vi "Read Waveform (Multiple).vi"(8 "error in (no error)":errorcluster, 9 "Maximum Time (10000 ms)":u32=10000, 10 "Channels":u16[](array[ring])=[1, 2] items=["Channel 1"=1, "Channel 2"=2], 11 "VISA resource name":refnum<visa-resource-name>) -> (0 "error out":errorcluster, 2 "Waveform Data":waveform(dbl)[](graph), 3 "VISA resource name out":refnum<visa-resource-name>)   [LabVIEW 2013, in "Template - Scope.lvlib"]
doc: "Initiates an acquisition on all channels that you enabled with the Configure Channel VI. The VI waits for the acquisition to complete and returns the waveform for the <B>Source Channel</B> you specified. If the oscilloscope did not complete the acquisition within the time period you specify with the <B>Timeout</B> control, the VI returns a timeout error. A common cause for a timeout error is the acquisition was not triggered. For example, the trigger level is out of range of the waveform. \n\n<B>Note:</B> If your instrument does not support auto compensation for probe attenuation, you may need to adjust the scaling of the waveform data accordingly. This is handled automatically in the Configure Channel VI or can be done manually by multiplying the waveform data by the probe attenuation."
uses:
  <instrlib>/_Template - Scope/Template - Scope.lvlib
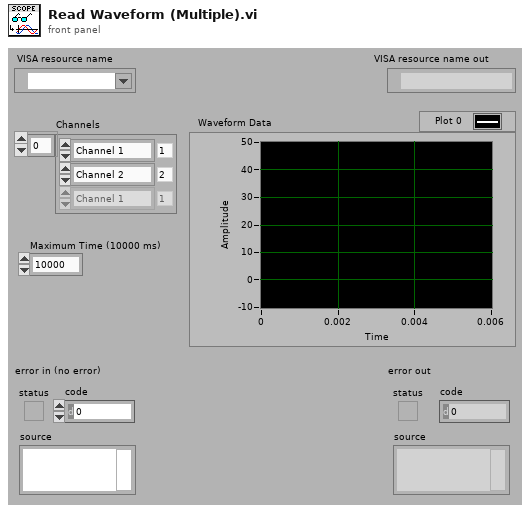
[diagram p1: front panel]
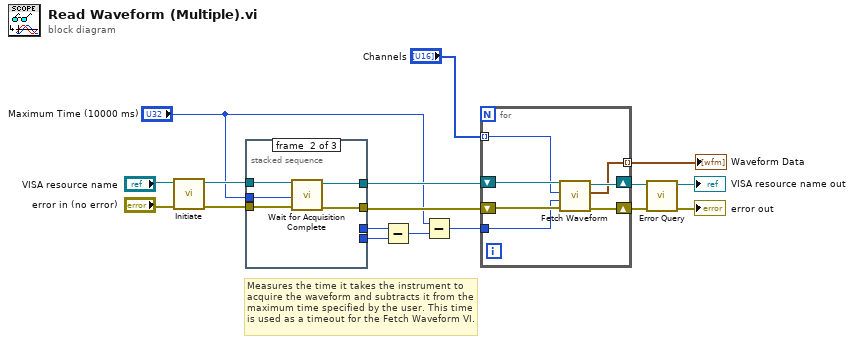
[diagram p0: block diagram]
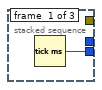
[diagram p2: hidden frame]
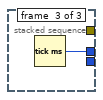
[diagram p3: hidden frame]
diagram:
  # "Measures the time it takes the instrument to acquire the waveform and subtracts it from the maximum time specified by the user. This time is used as a timeout for the Fetch Waveform VI."
  n1 = call <instrlib>:"Initiate.vi"("error in (no error)"="error in (no error)", "VISA resource name"="VISA resource name") -> ("error out"=w6:errorcluster, "VISA resource name out"=w5:refnum<visa-resource-name>)  [unwired: 8 in]
  n2 = stacked-sequence {
    tunnel: w5 -> [_ w23 _]
    tunnel: [_ w22 _] -> w4
    tunnel: w6 -> [_ w21 _]
    tunnel: [_ w20 _] -> w3
    tunnel: "Maximum Time (10000 ms)" -> [_ w19 _]
    tunnel: [w18 _ _] -> w8
    tunnel: [_ _ w24] -> w7
    frame #0 {
      n3 = Tick Count (ms)() -> (millisecond timer value=w18:u32)
    }
    frame #1 {
      n4 = call <instrlib>:"Wait for Acquisition Complete.vi"("error in (no error)"=w21, "Maximum Time (10000 ms)"=w19, "VISA resource name"=w23) -> ("error out"=w20:errorcluster, "VISA resource name out"=w22:refnum<visa-resource-name>)  [unwired: 7 in]
    }
    frame #2 {
      n5 = Tick Count (ms)() -> (millisecond timer value=w24:u32)
    }
  }
  n6 = Subtract(x=w7, y=w8) -> (x-y=w9:u32)
  n7 = Subtract(x="Maximum Time (10000 ms)", y=w9) -> (x-y=w2:u32)
  n8 = for {
    shift-right: [w30] -> w14
    shift-left: w3 -> [w28]
    tunnel: "Channels" -> [w27] mode=indexing
    tunnel: [w26] -> w10 mode=indexing
    shift-right: [w31] -> w15
    shift-left: w4 -> [w29]
    tunnel: w2 -> [w25]
    n9 = call <instrlib>:"Fetch Waveform.vi"("error in (no error)"=w28, "Timeout (10000 ms)"=w25, "Channel (1: Channel 1)"=w27, "VISA resource name"=w29) -> ("error out"=w30:errorcluster, "Waveform Data"=w26:waveform(dbl), "VISA resource name out"=w31:refnum<visa-resource-name>)  [unwired: 5 in]
  }
  "Waveform Data" <- w10
  n10 = call <instrlib>:"Error Query.vi"("error in (no error)"=w14, "VISA resource name"=w15) -> ("error out"=→"error out":errorcluster, "VISA resource name out"=→"VISA resource name out":refnum<visa-resource-name>)  [unwired: 6 in, 2 out]
